vi "test_AK RS-xxx Write.vi"(8 "error in (no error)":errorcluster, 11 "TestCase in":refnum<class "Serial Protocols Tests.lvclass">) -> (0 "error out":errorcluster, 3 "TestCase out":refnum<class "Serial Protocols Tests.lvclass">)   [LabVIEW 2019, in "Serial Protocols Tests.lvclass"]
uses:
  Serial Protocols Tests.lvclass
  Listener/Listener.lvclass
  Listener/ListenerClassControls/Operation.ctl
  AK RS-xxx/AK RS-xxx.lvclass
  D:/GitRepository/niveristand-instrument-addon-classes/Source/Protocols/Protocol Parent/Protocol Parent.lvclass
  D:/GitRepository/niveristand-instrument-addon-classes/Source/Protocols/RS-xxx/RS-xxx.lvclass
  <vilib>/Platform/TimedLoop/XDataNode/timing_clust.ctl
  <vilib>/Platform/TimedLoop/XDataNode/nitl_modes.ctl
  <vilib>/Platform/TimedLoop/XDataNode/wakeup.ctl
  RS-xxx/RS-xxx.lvclass/RS-xxx.ctl
  AK RS-xxx/AK RS-xxx.lvclass/AK RS-xxx.ctl
  Constants.vi
  <vilib>/platform/TimedLoop/XDataNode/XDataNode.xnode
  <vilib>/addons/_JKI Toolkits/VI Tester/TestCase.llb/TestCase.lvclass
  RS-xxx/RS-xxx.lvclass
  <vilib>/Platform/TimedLoop/XDataNode/XDNodeRunTimeDep.lvlib
  C:/Program Files (x86)/National Instruments/LabVIEW 2019/vi.lib/addons/_JKI Toolkits/VI Tester/TestCase.llb/TestCase.lvclass
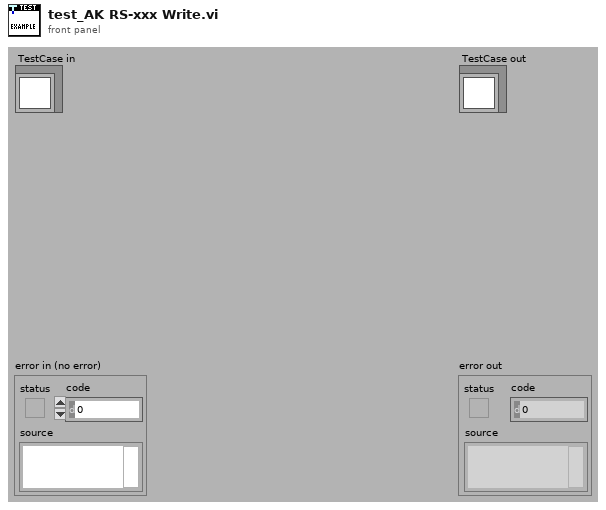
[diagram p1: front panel]
types:
  T1 = typedef "Listener.lvclass/Operation.ctl" = enum16{"Read", "Write"}
  T2 = typedef "XDNodeRunTimeDep.lvlib/timing_clust.ctl" = cluster{"Expected End [f-1]":u64, "Actual End [f-1]":u64, "Finished Late? [f-1]":bool, "Expected End [i-1]":u64, "Actual End [i-1]":u64, "Finished Late? [i-1]":bool, "Expected Start [i]":u64, "Actual Start [i]":u64, "Expected Start [f]":u64, "Actual Start [f]":u64, "Source Name":string, "Structure Name":string, "Period":i64, "Deadline":i64, "Offset":i64, "Start":i64, "Priority":i32, "Timeout":i32, "Mode":T3, "Wakeup Reason":T4, "Error":errorcluster, "Source Type":string, "Secondary Source Type":string, "Global End Time":u64, "Global Start Time":u64, "Frame Duration":u64, "Iteration Duration":u64, "Assigned CPU":i32, "I/O Scan Engine Mode":u32}
  T3 = typedef "XDNodeRunTimeDep.lvlib/nitl_modes.ctl" = enum32{"No Change", "Process missed periods, maintain original phase", "Discard missed periods, maintain original phase", "Process missed periods, ignore original phase", "Discard missed periods, ignore original phase"}
  T4 = typedef "XDNodeRunTimeDep.lvlib/wakeup.ctl" = enum32{"Normal", "Aborted", "Asynchronous wakeup", "Timing source error", "Timed loop error", "Timeout"}
  T5 = typedef "Listener.lvclass/RS-xxx Data Structure.ctl" = cluster{"Virtual COM Port Settings 1":cluster{"Port":string, "Baud Rate":u32, "Data Bits":u16, "Parity":enum16{"None", "Odd", "Even", "Mark", "Space"}, "Stop Bits":u16, "Flow Control":u16, "XON":enum16{"NUL", "SOH", "STX", "ETX", "EOT", "ENQ", "ACK", "BEL", "BS", "HT", "LF", "VT", "FF", "CR", "SO", "SI", "DLE", "DC1", "DC2", "DC3", "DC4", "NAK", "SYN", "ETB", "CAN", "EM", "SUB", "ESC", "FS", "GS", "RS", "US", "SP", "!", "\"", "#", "$", "%", "&", "'", "(", ")", "*", "+", ",", "- (-)", ".", "/", "0", "1", "2", "3", "4", "5", "6", "7", "8", "9", ":", ";", "<", "=", ">", "?", "@", "A", "B", "C", "D", "E", "F", "G", "H", "I", "J", "K", "L", "M", "N", "O", "P", "Q", "R", "S", "T", "U", "V", "W", "X", "Y", "Z", "[", "\\", "]", "^", "_", "`", "a", "b", "c", "d", "e", "f", "g", "h", "i", "j", "k", "l", "m", "n", "o", "p", "q", "r", "s", "t", "u", "v", "w", "x", "y", "z", "{", "|", "}", "~"}, "XOFF":enum16{"NUL", "SOH", "STX", "ETX", "EOT", "ENQ", "ACK", "BEL", "BS", "HT", "LF", "VT", "FF", "CR", "SO", "SI", "DLE", "DC1", "DC2", "DC3", "DC4", "NAK", "SYN", "ETB", "CAN", "EM", "SUB", "ESC", "FS", "GS", "RS", "US", "SP", "!", "\"", "#", "$", "%", "&", "'", "(", ")", "*", "+", ",", "- (-)", ".", "/", "0", "1", "2", "3", "4", "5", "6", "7", "8", "9", ":", ";", "<", "=", ">", "?", "@", "A", "B", "C", "D", "E", "F", "G", "H", "I", "J", "K", "L", "M", "N", "O", "P", "Q", "R", "S", "T", "U", "V", "W", "X", "Y", "Z", "[", "\\", "]", "^", "_", "`", "a", "b", "c", "d", "e", "f", "g", "h", "i", "j", "k", "l", "m", "n", "o", "p", "q", "r", "s", "t", "u", "v", "w", "x", "y", "z", "{", "|", "}", "~"}, "End Read on Termination Character":bool, "End Write on Termination Character":bool, "Termination Character":u8}, "Virtual COM Port Settings 2":cluster{"Port":string, "Baud Rate":u32, "Data Bits":u16, "Parity":enum16{"None", "Odd", "Even", "Mark", "Space"}, "Stop Bits":u16, "Flow Control":u16, "XON":enum16{"NUL", "SOH", "STX", "ETX", "EOT", "ENQ", "ACK", "BEL", "BS", "HT", "LF", "VT", "FF", "CR", "SO", "SI", "DLE", "DC1", "DC2", "DC3", "DC4", "NAK", "SYN", "ETB", "CAN", "EM", "SUB", "ESC", "FS", "GS", "RS", "US", "SP", "!", "\"", "#", "$", "%", "&", "'", "(", ")", "*", "+", ",", "- (-)", ".", "/", "0", "1", "2", "3", "4", "5", "6", "7", "8", "9", ":", ";", "<", "=", ">", "?", "@", "A", "B", "C", "D", "E", "F", "G", "H", "I", "J", "K", "L", "M", "N", "O", "P", "Q", "R", "S", "T", "U", "V", "W", "X", "Y", "Z", "[", "\\", "]", "^", "_", "`", "a", "b", "c", "d", "e", "f", "g", "h", "i", "j", "k", "l", "m", "n", "o", "p", "q", "r", "s", "t", "u", "v", "w", "x", "y", "z", "{", "|", "}", "~"}, "XOFF":enum16{"NUL", "SOH", "STX", "ETX", "EOT", "ENQ", "ACK", "BEL", "BS", "HT", "LF", "VT", "FF", "CR", "SO", "SI", "DLE", "DC1", "DC2", "DC3", "DC4", "NAK", "SYN", "ETB", "CAN", "EM", "SUB", "ESC", "FS", "GS", "RS", "US", "SP", "!", "\"", "#", "$", "%", "&", "'", "(", ")", "*", "+", ",", "- (-)", ".", "/", "0", "1", "2", "3", "4", "5", "6", "7", "8", "9", ":", ";", "<", "=", ">", "?", "@", "A", "B", "C", "D", "E", "F", "G", "H", "I", "J", "K", "L", "M", "N", "O", "P", "Q", "R", "S", "T", "U", "V", "W", "X", "Y", "Z", "[", "\\", "]", "^", "_", "`", "a", "b", "c", "d", "e", "f", "g", "h", "i", "j", "k", "l", "m", "n", "o", "p", "q", "r", "s", "t", "u", "v", "w", "x", "y", "z", "{", "|", "}", "~"}, "End Read on Termination Character":bool, "End Write on Termination Character":bool, "Termination Character":u8}, "Data":string, "Data Length":u32}
  T6 = cluster{"Port":string, "Baud Rate":u32, "Data Bits":u16, "Parity":enum16{"None", "Odd", "Even", "Mark", "Space"}, "Stop Bits":u16, "Flow Control":u16, "XON":enum16{"NUL", "SOH", "STX", "ETX", "EOT", "ENQ", "ACK", "BEL", "BS", "HT", "LF", "VT", "FF", "CR", "SO", "SI", "DLE", "DC1", "DC2", "DC3", "DC4", "NAK", "SYN", "ETB", "CAN", "EM", "SUB", "ESC", "FS", "GS", "RS", "US", "SP", "!", "\"", "#", "$", "%", "&", "'", "(", ")", "*", "+", ",", "- (-)", ".", "/", "0", "1", "2", "3", "4", "5", "6", "7", "8", "9", ":", ";", "<", "=", ">", "?", "@", "A", "B", "C", "D", "E", "F", "G", "H", "I", "J", "K", "L", "M", "N", "O", "P", "Q", "R", "S", "T", "U", "V", "W", "X", "Y", "Z", "[", "\\", "]", "^", "_", "`", "a", "b", "c", "d", "e", "f", "g", "h", "i", "j", "k", "l", "m", "n", "o", "p", "q", "r", "s", "t", "u", "v", "w", "x", "y", "z", "{", "|", "}", "~"}, "XOFF":enum16{"NUL", "SOH", "STX", "ETX", "EOT", "ENQ", "ACK", "BEL", "BS", "HT", "LF", "VT", "FF", "CR", "SO", "SI", "DLE", "DC1", "DC2", "DC3", "DC4", "NAK", "SYN", "ETB", "CAN", "EM", "SUB", "ESC", "FS", "GS", "RS", "US", "SP", "!", "\"", "#", "$", "%", "&", "'", "(", ")", "*", "+", ",", "- (-)", ".", "/", "0", "1", "2", "3", "4", "5", "6", "7", "8", "9", ":", ";", "<", "=", ">", "?", "@", "A", "B", "C", "D", "E", "F", "G", "H", "I", "J", "K", "L", "M", "N", "O", "P", "Q", "R", "S", "T", "U", "V", "W", "X", "Y", "Z", "[", "\\", "]", "^", "_", "`", "a", "b", "c", "d", "e", "f", "g", "h", "i", "j", "k", "l", "m", "n", "o", "p", "q", "r", "s", "t", "u", "v", "w", "x", "y", "z", "{", "|", "}", "~"}, "End Read on Termination Character":bool, "End Write on Termination Character":bool, "Termination Character":u8}
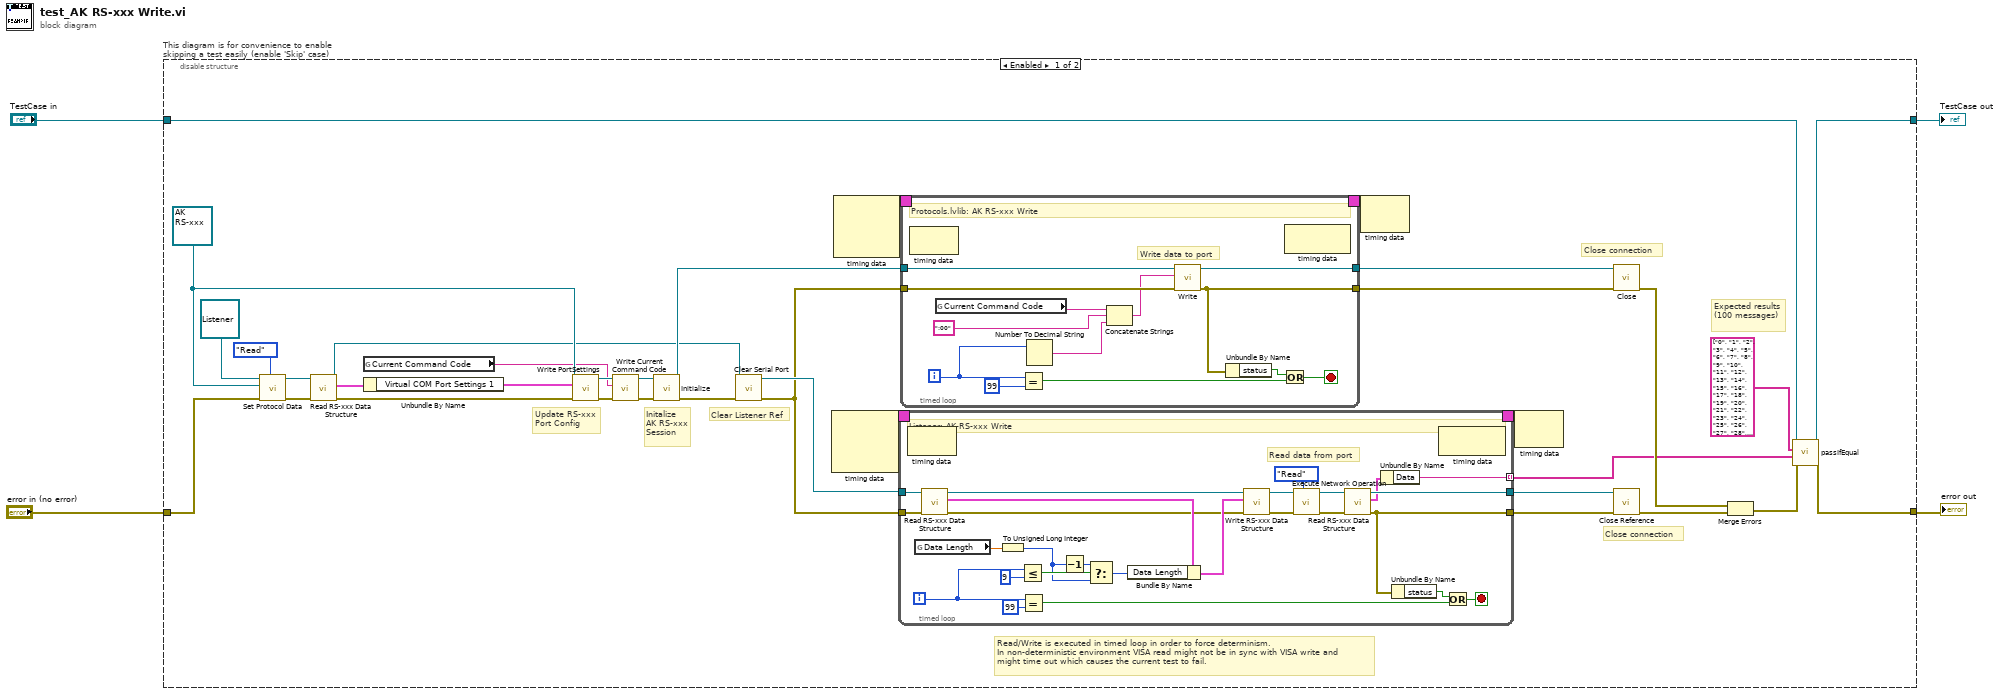
[diagram p0: block diagram]
diagram:
  n1 = disable-structure "This diagram is for convenience to enable skipping a test easily (enable 'Skip' case)" shown="Enabled" {
    disable-tunnel: "TestCase in" -> [w39 w90]
    disable-tunnel: [w38 w88] -> w1
    disable-tunnel: [w37 w89] -> w3
    disable-tunnel: "error in (no error)" -> [w36 w87]
    frame Enabled {
      w19 = refnum<class "AK RS-xxx.lvclass"> refnum ("Protocols.lvlib:AK RS-xxx.lvclass")
      # "Clear Listener Ref"
      # "Update RS-xxx \nPort Config"
      # "Initalize \nAK RS-xxx\nSession"
      # "Close connection"
      # "Close connection"
      # "Expected results\n(100 messages)"
      # "Read/Write is executed in timed loop in order to force determinism.\nIn non-deterministic environment VISA read might not be in sync with VISA write and\nmight time out which causes the current test to fail."
      n2 = call "Set Protocol Data.vi"("Operation"=Operation."Read", "error in (no error)"=w36, "Protocols.lvlib:Protocol Parent.lvclass"=w19, "Listener In.lvclass"=refnum<class "Listener.lvclass"> refnum ("Listener.lvclass")) -> ("error out"=w22:errorcluster, "Listener Out.lvclass"=w23:refnum<class "Listener.lvclass">)  [unwired: 6 in]
      n3 = call-dynamic "Read RS-xxx Data Structure.vi"("error in (no error)"=w22, "Listener in"=w23) -> ("error out"=w10:errorcluster, "RS-xxx Data Structure"=w20:T5, "Listener out"=w7:refnum<class "Listener.lvclass">)  [unwired: 7 in]
      n4 = global read "Constants.vi" "Current Command Code"() -> (w15:string)
      n5 = Unbundle By Name(w20) -> ("Virtual COM Port Settings 1"=w18:T6)
      n6 = call "Write PortSettings.vi"("error in (no error)"=w10, "Cluster"=w18, "RS232 in"=w19) -> ("error out"=w16:errorcluster, "RS232 out"=w17:refnum<class "AK RS-xxx.lvclass">)  [unwired: 7 in]
      n7 = call "Write Current Command Code.vi"("error in (no error)"=w16, "Current Command Code"=w15, "AK RS232 in"=w17) -> ("error out"=w9:errorcluster, "AK RS232 out"=w14:refnum<class "AK RS-xxx.lvclass">)  [unwired: 7 in]
      n8 = call-dynamic "Initialize.vi"("error in (no error)"=w9, "RS232 in"=w14) -> ("error out"=w8:errorcluster, "RS232 out"=w21:refnum<class "AK RS-xxx.lvclass">)  [unwired: 8 in]
      n9 = call "Clear Serial Port.vi"("error in (no error)"=w8, "Listener In.lvclass"=w7) -> ("error out"=w5:errorcluster, "Listener out"=w6:refnum<class "Listener.lvclass">)  [unwired: 8 in]
      n10 = node-c288() -> (w35:T2)  [unwired: 3 in]
      n11 = node-c288() -> (w33:T2)  [unwired: 3 in]
      n12 = timed-loop {
        timing: w35 -> [_]
        timing-out: [_] -> w34
        tunnel: [w74] -> w12 mode=indexing
        tunnel: w5 -> [w66]
        tunnel: [w58] -> w24
        tunnel: w6 -> [w67]
        tunnel: [w76] -> w25
        i -> [w70]
        stop <- w80 stop-if-true
        # "Read data from port"
        # "Listener: AK-RS-xxx Write"
        n13 = node-c288() -> ()  [unwired: 1 in, 1 out]
        n14 = global read "Constants.vi" "Data Length"() -> (w69:dbl)
        n15 = call-dynamic "Read RS-xxx Data Structure.vi"("error in (no error)"=w66, "Listener in"=w67) -> ("error out"=w59:errorcluster, "RS-xxx Data Structure"=w64:T5, "Listener out"=w63:refnum<class "Listener.lvclass">)  [unwired: 7 in]
        n16 = To Unsigned Long Integer(number=w69) -> (unsigned 32bit integer=w68:u32)
        n17 = Less Or Equal?(x=w70, y=9) -> (x <= y?=w72:bool)
        n18 = Equal?(x=w70, y=99) -> (x = y?=w81:bool)
        n19 = Decrement(x=w68) -> (x-1=w71:u32)
        n20 = Select(t=w71, s=w72, f=w68) -> (s? t:f=w65:u32)
        n21 = Bundle By Name(cluster=w64, "Data Length"=w65) -> (w60:T5)
        n22 = call-dynamic "Write RS-xxx Data Structure.vi"("error in (no error)"=w59, "RS-xxx Data Structure"=w60, "Listener in"=w63) -> ("error out"=w61:errorcluster, "Listener out"=w62:refnum<class "Listener.lvclass">)  [unwired: 7 in]
        n23 = call "Execute Network Operation.vi"("Operation"=Operation."Read", "error in (no error)"=w61, "Listener In.lvclass"=w62) -> ("error out"=w78:errorcluster, "Listener Out.lvclass"=w77:refnum<class "Listener.lvclass">)  [unwired: 7 in]
        n24 = call-dynamic "Read RS-xxx Data Structure.vi"("error in (no error)"=w78, "Listener in"=w77) -> ("error out"=w58:errorcluster, "RS-xxx Data Structure"=w75:T5, "Listener out"=w76:refnum<class "Listener.lvclass">)  [unwired: 7 in]
        n25 = Unbundle By Name(w75) -> ("Data"=w74:string)
        n26 = Unbundle By Name(w58) -> ("status"=w57:bool)
        n27 = node-c288() -> ()  [unwired: 1 in, 1 out]
        n28 = Or(x=w57, y=w81) -> (x .or. y?=w80:bool)
      }
      n29 = timed-loop {
        timing: w33 -> [_]
        timing-out: [_] -> w32
        tunnel: w21 -> [w48]
        tunnel: [w47] -> w13
        tunnel: w5 -> [w49]
        tunnel: [w41] -> w26
        i -> [w46]
        stop <- w50 stop-if-true
        # "Write data to port"
        # "Protocols.lvlib: AK RS-xxx Write"
        n30 = node-c288() -> ()  [unwired: 1 in, 1 out]
        n31 = global read "Constants.vi" "Current Command Code"() -> (w44:string)
        n32 = Equal?(x=w46, y=99) -> (x = y?=w52:bool)
        n33 = Number To Decimal String(number=w46) -> (decimal integer string=w43:string)  [unwired: 1 in]
        n34 = Concatenate Strings(w44, ":00", w43) -> (w42:string)
        n35 = call-dynamic "Write.vi"("error in (no error)"=w49, "String"=w42, "AK RS232 in"=w48) -> ("error out"=w41:errorcluster, "AK RS232 out"=w47:refnum<class "AK RS-xxx.lvclass">)  [unwired: 7 in]
        n36 = Unbundle By Name(w41) -> ("status"=w40:bool)
        n37 = Or(x=w40, y=w52) -> (x .or. y?=w50:bool)
        n38 = node-c288() -> ()  [unwired: 1 in, 1 out]
      }
      n39 = node-c288(w32) -> ()  [unwired: 1 out]
      n40 = node-c288(w34) -> ()  [unwired: 1 out]
      n41 = call-dynamic "Close.vi"("error in (no error)"=w26, "RS232 in"=w13) -> ("error out"=w28:errorcluster)  [unwired: 8 in, 1 out]
      n42 = call "Close Reference.vi"("error in (no error)"=w24, "Listener In.lvclass"=w25) -> ("error out"=w27:errorcluster)  [unwired: 9 in]
      n43 = Merge Errors(w28, w27) -> (w29:errorcluster)
      n44 = call-dynamic "passIfEqual.vi"("error in (no error)"=w29, "y"=w12, "x"=string[] ["0", "1", "2", "3", "4", "5", "6", "7", "8", "9", "10", "11", "12", "13", "14", "15", "16", "17", "18", "19", "20", "21", "22", "23", "24", "25", "26", "27", "28", "29", "30", "31", "32", "33", "34", "35", "36", "37", "38", "39", "40", "41", "42", "43", "44", "45", "46", "47", "48", "49", "50", "51", "52", "53", "54", "55", "56", "57", "58", "59", "60", "61", "62", "63", "64", "65", "66", "67", "68", "69", "70", "71", "72", "73", "74", "75", "76", "77", "78", "79", "80", "81", "82", "83", "84", "85", "86", "87", "88", "89", "90", "91", "92", "93", "94", "95", "96", "97", "98", "99"] ("Array"), "TestCase in"=w39) -> ("error out"=w37:errorcluster, "TestCase out"=w38:refnum<class "Serial Protocols Tests.lvclass">)  [unwired: 6 in]
    }
    frame Disabled {
      # "skip test result while test is under development"
      n45 = call <vilib>:"skip.vi"("error in (no error)"=w87, "TestCase in"=w90) -> ("error out"=w89:errorcluster, "TestCase out"=w88:refnum<class "Serial Protocols Tests.lvclass">)  [unwired: 8 in]
    }
  }
  "error out" <- w3
  "TestCase out" <- w1
